vi "Anritsu VNA Set Stimulus.vi"(7 "Anritsu VNA":T4={"Model"="8753C", "Serial"="", "Firmware"="", "Learn String"=""}, 8 "error in (no error)":errorcluster, 9 "Channel":i8=1 min=1 max=99 step=1, 10 "Stimulus":T1={"Use Instrument Settings"=FALSE, "Blank Frequencies"=FALSE, "Sweep Type"=enum."Linear", "Sweep"={"Fstart"=500.0, "Fstop"=1500.0, "Units"=enum."MHz", "Points"=201}, "Power (dBm)"=999.0, "IFBW (Hz)"=-1.0, "Sweep Time (s)"=-1.0, "Calibration"={"State"=FALSE, "String"=""}} {"Sweep Time (s)" format="%.3g"}, 11 "VISA Resource Name":refnum<visa-resource-name>) -> (0 "error out":errorcluster {"code" format="%.0x"}, 3 "dup VISA Resource Name":refnum<visa-resource-name>)   [LabVIEW 2011]
uses:
  TypeDefs/Anritsu VNA Instrument Info.ctl
  tests/S Parameter/TypeDefs/SP Stimulus Parameters.ctl
  tests/S Parameter/TypeDefs/SP Frequency Units.ctl
  tests/S Parameter/TypeDefs/SP Calibration State.ctl
  TypeDefs/Anritsu VNA Sweep Type.ctl
  TypeDefs/Anritsu VNA Trigger Mode.ctl
panel:
  in  "Case Constant":bool
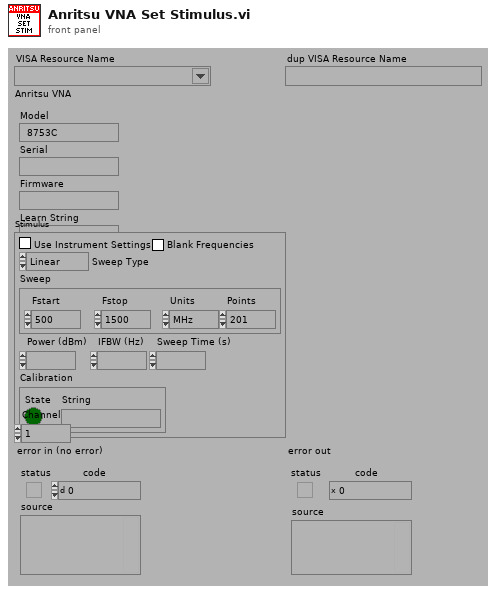
[diagram p1: front panel]
types:
  T1 = typedef "SP Stimulus Parameters.ctl" = cluster{"Use Instrument Settings":bool, "Blank Frequencies":bool, "Sweep Type":enum32{"Linear", "Logarithmic", "List", "Power", "CW"}, "Sweep":cluster{"Fstart":dbl, "Fstop":dbl, "Units":T2, "Points":i32}, "Power (dBm)":dbl, "IFBW (Hz)":dbl, "Sweep Time (s)":dbl, "Calibration":T3}
  T2 = typedef "SP Frequency Units.ctl" = enum16{"Hz", "kHz", "MHz", "GHz", "Points"}
  T3 = typedef "SP Calibration State.ctl" = cluster{"State":bool, "String":string}
  T4 = typedef "Anritsu VNA Instrument Info.ctl" = cluster{"Model":string, "Serial":string, "Firmware":string, "Learn String":string}
  T5 = typedef "Anritsu VNA Sweep Type.ctl" = enum32{"Linear Sweep", "Frequency Sweep", "Power Sweep", "CW Time Sweep", "Discrete Fill", "Time Domain", "Logarithmic Sweep", "Segmented Sweep (Frequency)", "Segmented Sweep (Index)", "MFGC"}
  T6 = typedef "Anritsu VNA Trigger Mode.ctl" = enum16{"Continuous", "Hold", "Single"}
  T7 = cluster{"Converted Frequency":dbl, "Converted Frequency":dbl}
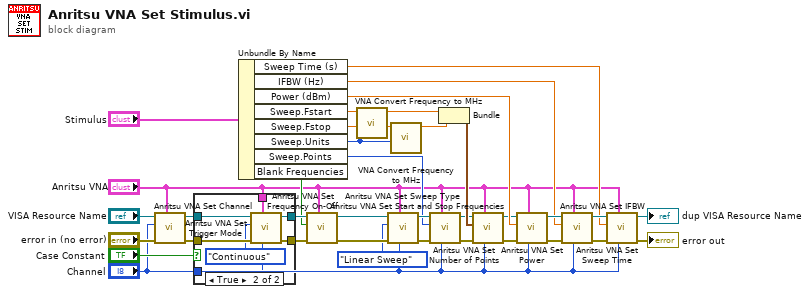
[diagram p0: block diagram]
diagram:
  n1 = call "Anritsu VNA Set Channel.vi"("Anritsu VNA"="Anritsu VNA", "error in (no error)"="error in (no error)", "Channel"="Channel", "VISA Resource Name"="VISA Resource Name") -> ("error out"=w2:errorcluster, "dup VISA Resource Name"=w3:refnum<visa-resource-name>)  [unwired: 6 out]
  n2 = case shown="True" "Case Constant" {
    tunnel: [w38 w42] -> w28
    tunnel: [w37 w43] -> w27
    tunnel: w2 -> [w38 w45]
    tunnel: w3 -> [w37 w44]
    tunnel: "Anritsu VNA" -> [_ w40]
    tunnel: "Channel" -> [_ w39]
    frame False {
    }
    frame True {
      n3 = call "Anritsu VNA Set Trigger Mode.vi"("Channel"=w39, "Anritsu VNA"=w40, "error in (no error)"=w45, "Trigger Mode"=Anritsu_VNA_Trigger_Mode."Continuous", "VISA Resource Name"=w44) -> ("error out"=w42:errorcluster, "dup VISA Resource Name"=w43:refnum<visa-resource-name>)  [unwired: 5 out]
    }
  }
  n4 = Unbundle By Name("Stimulus") -> ("Sweep Time (s)"=w13:dbl, "IFBW (Hz)"=w14:dbl, "Power (dBm)"=w35:dbl, "Sweep.Fstart"=w11:dbl, "Sweep.Fstop"=w10:dbl, "Sweep.Units"=w7:T2, "Sweep.Points"=w12:i32, "Blank Frequencies"=w24:bool)
  n5 = call "Anritsu VNA Set Frequency On-Off.vi"("Anritsu VNA"="Anritsu VNA", "error in (no error)"=w28, "Blank Frequencies (F)"=w24, "VISA Resource Name"=w27) -> ("error out"=w25:errorcluster, "dup VISA Resource Name"=w26:refnum<visa-resource-name>)  [unwired: 6 out]
  n6 = call "VNA Convert Frequency to MHz.vi"("Units"=w7, "Frequency"=w11) -> ("Converted Frequency"=w8:dbl)  [unwired: 9 out]
  n7 = call "Anritsu VNA Set Sweep Type.vi"("Channel"="Channel", "Anritsu VNA"="Anritsu VNA", "error in (no error)"=w25, "Sweep Type"=Anritsu_VNA_Sweep_Type."Linear Sweep", "VISA Resource Name"=w26) -> ("error out"=w29:errorcluster, "dup VISA Resource Name"=w30:refnum<visa-resource-name>)  [unwired: 5 out]
  n8 = call "VNA Convert Frequency to MHz.vi"("Units"=w7, "Frequency"=w10) -> ("Converted Frequency"=w9:dbl)  [unwired: 9 out]
  n9 = call "Anritsu VNA Set Number of Points.vi"("Channel"="Channel", "Anritsu VNA"="Anritsu VNA", "error in (no error)"=w29, "Number Points"=w12, "VISA Resource Name"=w30) -> ("error out"=w31:errorcluster, "dup VISA Resource Name"=w32:refnum<visa-resource-name>)  [unwired: 5 out]
  n10 = Bundle("Converted Frequency"=w8, "Converted Frequency"=w9) -> (w33:T7)  [unwired: 1 out]
  n11 = call "Anritsu VNA Set Start and Stop Frequencies.vi"("Channel"="Channel", "Anritsu VNA"="Anritsu VNA", "error in (no error)"=w31, "Start/Stop Freqs, MHz"=w33, "VISA Resource Name"=w32) -> ("error out"=w21:errorcluster, "dup VISA Resource Name"=w22:refnum<visa-resource-name>)  [unwired: 1 in, 4 out]
  n12 = call "Anritsu VNA Set Power.vi"("Channel"="Channel", "Anritsu VNA"="Anritsu VNA", "error in (no error)"=w21, "Source Power, dBm (0.0)"=w35, "VISA Resource Name"=w22) -> ("error out"=w15:errorcluster, "dup VISA Resource Name"=w20:refnum<visa-resource-name>)  [unwired: 5 out]
  n13 = call "Anritsu VNA Set IFBW.vi"("Channel"="Channel", "Anritsu VNA"="Anritsu VNA", "error in (no error)"=w15, "IFBW, Hz (3000)"=w14, "VISA Resource Name"=w20) -> ("error out"=w16:errorcluster, "dup VISA Resource Name"=w19:refnum<visa-resource-name>)  [unwired: 5 out]
  n14 = call "Anritsu VNA Set Sweep Time.vi"("Channel"="Channel", "Anritsu VNA"="Anritsu VNA", "error in (no error)"=w16, "Sweep Time, s (-1: Auto)"=w13, "VISA Resource Name"=w19) -> ("error out"=→"error out":errorcluster, "dup VISA Resource Name"=→"dup VISA Resource Name":refnum<visa-resource-name>)  [unwired: 5 out]
